vi "Day 2 Task 2.vi"() -> ()   [LabVIEW 2018]
panel:
  out "aim":i64
  out "Horizontal * vertical (multiplied)":i64
  out "vertical position":i64
  out "horizontal position":i64
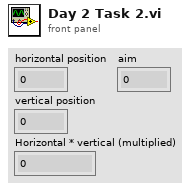
[diagram p1: front panel]
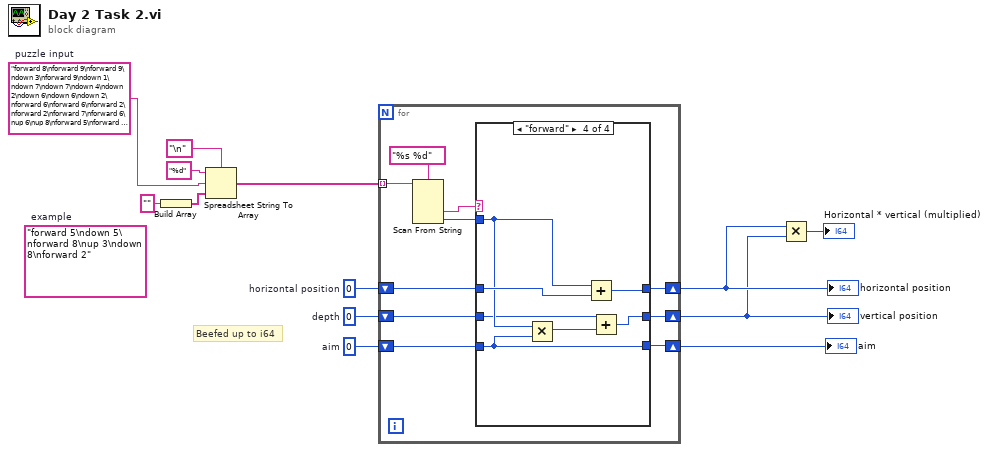
[diagram p0: block diagram]
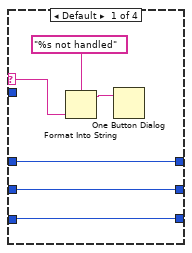
[diagram p2: hidden frame]
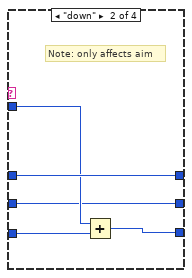
[diagram p3: hidden frame]
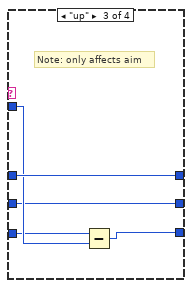
[diagram p4: hidden frame]
diagram:
  w3 = i64 0  # aim
  w1 = "forward 8\nforward 9\nforward 9\ndown 3\nforward 9\ndown 1\ndown 7\ndown 7\ndown 4\ndown 2\ndown 6\ndown 6\ndown 2\nforward 6\nforward 6\nforward 2\nforward 2\nforward 7\nforward 6\nup 6\nup 8\nforward 5\nforward 4\ndown 6\nforward 7\ndown 5\nforward 5\ndown 8\ndown 8\ndown 7\nforward 4\ndown 2\nforward 7\nup 8\nforward 3\ndown 2\nforward 1\nup 3\nforward 3\nup 1\ndown 3\nup 7\nup 2\ndown 4\ndown 2\nforward 9\nforward 3\ndown 8\nforward 5\nup 9\nup 4\nforward 9\ndown 1\nforward 6\ndown 3\nforward 8\nup 2\nforward 3\nup 7\ndown 4\nforward 2\nforward 7\nforward 3\ndown 1\ndown 3\nup 5\nforward 6\ndown 5\ndown 4\ndown 8\ndown 2\nup 5\nforward 7\nup 8\nforward 2\ndown 5\nforward 3\nup 1\nup 5\ndown 8\ndown 3\nforward 4\nforward 4\nforward 1\nup 8\ndown 9\nforward 7\nforward 9\ndown 5\nup 3\ndown 9\nup 6\nforward 1\nforward 3\nforward 5\ndown 5\nforward 6\ndown 3\ndown 8\nforward 3\nforward 5\nforward 7\nforward 6\ndown 9\ndown 5\ndown 6\ndown 5\ndown 1\ndown 8\nforward 3\ndown 9\ndown 5\ndown 5\nforward 9\nforward 2\ndown 7\nforward 9\nforward 9\nup 1\nforward 3\nup 9\nforward 5\nforward 7\ndown 7\nforward 2\nup 8\nup 6\ndown 7\ndown 3\ndown 5\ndown 2\nforward 6\nforward 6\nup 6\nup 2\nforward 4\nforward 7\nforward 1\ndown 4\nup 8\ndown 3\nup 1\ndown 2\nforward 4\nforward 7\nup 1\ndown 7\nforward 8\nup 2\ndown 8\nup 4\nup 4\nup 2\ndown 8\nup 4\ndown 6\nup 8\ndown 5\nup 5\ndown 8\nforward 9\ndown 1\ndown 5\nforward 3\nforward 3\nup 9\ndown 2\nforward 3\ndown 6\nforward 1\nforward 9\nforward 3\ndown 8\nup 4\ndown 1\ndown 8\nup 1\nforward 2\ndown 7\nup 3\nup 8\ndown 2\nup 6\nforward 6\ndown 9\nforward 4\nforward 7\nup 9\nforward 3\nforward 2\ndown 8\ndown 2\ndown 5\ndown 5\ndown 1\nup 7\ndown 4\nforward 5\ndown 9\ndown 5\ndown 1\ndown 6\nforward 9\ndown 6\nforward 3\ndown 3\nup 6\nforward 2\nforward 6\ndown 2\ndown 9\ndown 6\ndown 1\ndown 7\ndown 6\ndown 6\nup 1\nforward 8\ndown 9\ndown 6\ndown 8\ndown 8\ndown 6\ndown 3\nforward 9\nforward 6\ndown 9\nforward 5\ndown 6\ndown 6\ndown 9\ndown 7\ndown 3\nforward 1\nup 9\nforward 9\ndown 7\nforward 4\ndown 1\nforward 9\nup 9\ndown 7\nforward 5\ndown 3\nup 7\nforward 9\nforward 6\nforward 3\nforward 8\ndown 4\ndown 1\ndown 7\ndown 7\nup 4\ndown 9\nforward 6\nforward 7\ndown 8\nforward 2\nforward 2\nforward 9\nforward 6\nforward 9\nup 6\nup 8\nforward 2\nup 3\nforward 9\nforward 1\ndown 4\nforward 8\ndown 4\nforward 5\nforward 7\nup 2\nforward 5\ndown 4\nforward 3\ndown 5\nforward 9\nup 3\nforward 8\ndown 7\ndown 7\ndown 9\nforward 2\ndown 1\ndown 6\nup 8\ndown 2\ndown 1\nup 3\ndown 3\nforward 2\nforward 6\nup 6\ndown 3\nup 9\nup 3\ndown 8\nup 6\ndown 2\nforward 4\nup 1\ndown 5\ndown 4\nup 9\nup 7\nforward 7\ndown 9\nforward 9\nforward 5\nforward 3\ndown 4\nup 6\nup 7\ndown 7\ndown 6\nup 9\nup 4\ndown 7\nforward 7\nforward 8\ndown 9\nforward 5\nforward 4\ndown 5\nforward 8\nforward 5\nup 3\ndown 9\nforward 1\nforward 2\nup 3\ndown 2\ndown 1\nforward 5\nforward 5\nforward 6\nup 2\nforward 3\ndown 7\ndown 6\nup 3\ndown 4\ndown 4\nforward 5\ndown 3\nup 6\nforward 1\nup 8\nforward 7\nforward 1\nforward 9\ndown 2\nup 8\nup 1\nup 4\nforward 9\nforward 3\nforward 5\ndown 1\nup 9\ndown 1\nforward 3\ndown 6\ndown 8\nup 4\nforward 6\nup 7\ndown 8\nforward 9\nup 2\ndown 7\ndown 1\nforward 9\nup 7\nforward 3\nforward 9\nforward 1\nforward 1\ndown 9\nforward 1\nup 4\ndown 5\nforward 4\ndown 1\nforward 4\nforward 9\nup 4\ndown 3\ndown 6\nup 2\ndown 6\ndown 5\nforward 5\nup 1\nup 9\nforward 8\nup 3\ndown 1\nforward 3\nforward 7\nup 6\nup 3\ndown 6\nforward 7\nup 6\ndown 7\nforward 8\nup 4\ndown 8\nup 9\nup 3\ndown 3\nforward 8\ndown 4\ndown 9\nforward 2\ndown 7\nup 1\nforward 9\nforward 5\nup 8\nforward 9\nforward 4\nforward 9\nforward 7\ndown 4\nup 4\ndown 7\ndown 4\ndown 4\ndown 1\nforward 5\nforward 4\ndown 1\ndown 4\ndown 8\ndown 3\nforward 7\nforward 4\ndown 1\ndown 9\nup 3\nforward 2\ndown 8\ndown 9\ndown 2\ndown 5\nup 9\ndown 9\nup 9\nforward 5\nforward 8\nforward 9\ndown 5\nforward 6\ndown 8\ndown 9\nforward 8\nup 5\nup 9\nup 7\nup 8\nforward 9\nforward 1\nup 6\ndown 8\ndown 8\nforward 1\nup 1\nforward 8\nforward 6\ndown 4\nforward 1\ndown 7\nforward 8\nforward 3\nup 3\ndown 4\ndown 2\nforward 2\nforward 3\nup 4\ndown 3\nforward 2\ndown 8\nforward 7\nup 3\ndown 2\nforward 2\ndown 5\nup 6\nup 6\nforward 4\nup 4\ndown 8\nforward 8\ndown 9\ndown 9\ndown 6\ndown 2\nforward 2\nup 6\nup 5\nforward 3\nforward 3\nup 9\ndown 3\nforward 8\ndown 5\nforward 5\nforward 7\ndown 3\ndown 4\ndown 1\ndown 8\ndown 1\ndown 1\nforward 9\nforward 3\ndown 8\ndown 6\nup 9\nforward 1\nforward 5\nup 9\nup 8\nforward 2\nup 8\ndown 9\nup 2\nforward 5\nforward 1\nforward 8\ndown 3\nforward 4\ndown 5\nup 6\nforward 8\nforward 9\nforward 3\ndown 1\ndown 3\ndown 3\nup 4\nforward 9\ndown 3\ndown 6\nforward 3\nforward 2\ndown 6\ndown 8\nforward 6\nup 8\nup 3\nup 4\nforward 2\nforward 4\nforward 4\nforward 7\ndown 6\nup 8\ndown 3\nforward 8\nforward 4\ndown 7\ndown 5\nforward 6\nforward 4\nforward 6\ndown 3\nforward 3\ndown 1\ndown 7\nforward 3\nforward 2\nforward 7\ndown 5\nup 4\ndown 6\ndown 9\nforward 3\nforward 5\nforward 3\ndown 1\nforward 2\nup 5\nup 6\nforward 2\ndown 4\nforward 3\ndown 4\ndown 1\nforward 8\nup 2\ndown 3\ndown 6\nup 5\nforward 3\nforward 6\ndown 3\nforward 1\ndown 7\nforward 2\nforward 1\nforward 6\nforward 5\nforward 3\ndown 4\ndown 8\nforward 1\nup 2\nup 8\ndown 4\nforward 9\nup 6\nforward 5\nforward 7\ndown 5\nforward 5\ndown 1\nforward 4\nforward 5\nup 2\nforward 5\nup 8\nup 1\nforward 2\ndown 4\ndown 6\nforward 4\ndown 2\ndown 3\nforward 2\nup 3\nup 4\nforward 2\ndown 6\nforward 1\nforward 4\ndown 6\nforward 7\nup 2\nforward 7\nforward 6\nup 2\nforward 8\nforward 4\nforward 9\ndown 1\ndown 8\nforward 3\nforward 2\ndown 8\nup 1\nforward 4\ndown 8\nforward 2\nforward 8\nup 2\ndown 1\nforward 4\nforward 2\nup 4\nup 2\ndown 3\nup 8\nforward 3\nup 8\nforward 9\nup 1\nup 5\ndown 5\ndown 6\nforward 1\nup 5\nup 8\nforward 7\ndown 5\nup 4\nforward 2\nup 4\nup 4\ndown 2\nforward 6\nforward 2\ndown 7\ndown 5\nforward 1\ndown 2\ndown 5\ndown 7\nup 8\ndown 8\nup 5\ndown 1\nforward 5\ndown 2\nforward 5\ndown 1\nup 7\nup 2\nforward 2\nforward 3\nforward 6\nforward 3\ndown 8\nup 8\nforward 8\nforward 1\nforward 7\nup 2\nforward 9\ndown 1\nforward 5\nup 9\nforward 3\nforward 7\nforward 8\nup 1\ndown 3\nforward 5\ndown 2\nforward 6\nforward 3\ndown 9\nup 5\nforward 2\ndown 4\nup 1\nforward 4\nup 4\ndown 8\ndown 8\nforward 3\nforward 8\ndown 7\nup 3\nforward 1\nup 3\nforward 9\nforward 7\nforward 1\ndown 6\nforward 3\ndown 1\ndown 8\nforward 5\nforward 3\nup 6\nforward 5\nforward 4\nforward 3\nforward 9\nforward 8\ndown 6\ndown 2\nforward 7\nforward 6\nup 6\ndown 6\ndown 4\ndown 3\nforward 8\ndown 9\nup 5\nforward 3\nforward 2\ndown 5\nup 4\ndown 6\ndown 3\nforward 9\ndown 2\nforward 9\nforward 8\nup 1\ndown 2\nforward 7\nup 5\nup 6\ndown 8\nup 9\nup 8\nforward 1\nforward 5\ndown 9\nforward 8\ndown 8\nup 1\ndown 7\nforward 7\nup 3\ndown 3\ndown 1\nforward 2\ndown 3\nforward 9\nforward 2\ndown 8\ndown 2\nforward 5\ndown 9\ndown 1\ndown 5\ndown 6\nup 4\nup 3\ndown 1\nup 7\nforward 6\ndown 3\ndown 6\nup 5\nforward 8\nup 8\ndown 1\ndown 2\nup 8\ndown 7\nforward 7\nforward 4\ndown 8\ndown 3\nforward 3\ndown 4\nforward 3\ndown 6\nforward 4\nforward 7\nforward 9\nup 7\nforward 1\ndown 7\ndown 8\ndown 8\nup 6\ndown 3\nforward 5\nforward 5\nforward 9\nforward 4\ndown 4\ndown 8\ndown 7\ndown 1\nforward 2\nforward 4\ndown 3\ndown 6\ndown 7\nforward 5\ndown 8\ndown 1\nforward 4\nforward 3\nforward 1\ndown 6\ndown 7\ndown 1\nforward 6\ndown 4\nup 2\nforward 4\ndown 2\nup 5\ndown 2\ndown 6\nup 7\nforward 4\nforward 7\nforward 9\nup 5\ndown 9\nup 5\nforward 6\ndown 2\nup 8\nup 9\nup 9\nforward 5\ndown 2\nforward 2\ndown 7\nforward 5\nforward 9\nup 8\ndown 8\nforward 1\ndown 2\nup 3\nforward 3\ndown 5\nforward 4\ndown 3\nforward 4\nforward 9\nforward 3\ndown 5\nforward 4\ndown 2\nforward 5\nforward 8\nup 6\nup 2\ndown 3\nforward 6\ndown 5\ndown 4\ndown 4\ndown 4\nup 2\nup 2\nforward 6\nforward 2\nforward 9\ndown 2\ndown 9\ndown 8\nforward 2\ndown 3\nup 3\nforward 5\ndown 4\nup 3\nforward 3\ndown 1\nforward 7\nforward 5\nforward 6\ndown 8\ndown 5\ndown 5\ndown 9\nup 2\nforward 3\ndown 4\ndown 9\nforward 3\nforward 9\nforward 2\nforward 4\nup 6\ndown 6\nup 9\nforward 8\ndown 7\nforward 1\nforward 4\nup 1\nup 2\ndown 9\nforward 6\ndown 6\ndown 1\ndown 4\ndown 7\ndown 6\nforward 5\nup 1\nup 7\ndown 2\ndown 8\ndown 2\ndown 7\ndown 3\nup 9\ndown 7\ndown 5\ndown 6\nforward 9\nup 3\nforward 2\ndown 8\nforward 4\ndown 6\nforward 3\nup 3\ndown 5\nup 4\nforward 6\nforward 7\nforward 9\ndown 3\nforward 7\nforward 3\ndown 4\nup 4\ndown 8\nforward 6\nforward 7\nforward 9\nforward 4\ndown 3\nup 5\ndown 7\ndown 7\nforward 9"  # puzzle input
  w7 = i64 0  # depth
  w8 = i64 0  # horizontal position
  (unwired) "forward 5\ndown 5\nforward 8\nup 3\ndown 8\nforward 2"  # example
  # "Beefed up to i64"
  n1 = Build Array("") -> (w11:string[])
  n2 = Spreadsheet String To Array(delimiter (Tab)="\n", format string="%d", spreadsheet string=w1, array type (2D Dbl)=w11) -> (array=w9:string[])
  n3 = for {
    tunnel: w9 -> [w21] mode=indexing
    shift-right: [w20] -> w6
    shift-left: w8 -> [w19]
    shift-right: [w17] -> w5
    shift-left: w7 -> [w18]
    shift-right: [w14] -> w2
    shift-left: w3 -> [w15]
    n4 = Scan From String(format string="%s %d", input string=w21) -> (output 1=w22:string, output 2=w16:i32)  [unwired: 4 in, 3 out]
    n5 = case shown="\"forward\"" w22 {
      selector: w22 -> [w27 _ _ _]
      tunnel: [w29 w34 w39 w45] -> w20
      tunnel: w19 -> [w29 w34 w39 w46]
      tunnel: w18 -> [w28 w30 w35 w41]
      tunnel: [w28 w30 w35 w40] -> w17
      tunnel: w16 -> [_ w33 w38 w43]
      tunnel: w15 -> [w24 w32 w37 w44]
      tunnel: [w24 w31 w36 w44] -> w14
      frame Default {
        n6 = Format Into String(format string="%s not handled", w27) -> (resulting string=w26:string)  [unwired: 2 in, 1 out]
        n7 = One Button Dialog(message=w26) -> ()  [unwired: 1 in, 1 out]
      }
      frame "down" {
        # "Note: only affects aim"
        n8 = Add(x=w33, y=w32) -> (x+y=w31:i64)
      }
      frame "up" {
        # "Note: only affects aim"
        n9 = Subtract(x=w37, y=w38) -> (x-y=w36:i64)
      }
      frame "forward" {
        n10 = Multiply(x=w43, y=w44) -> (x*y=w42:i64)
        n11 = Add(x=w43, y=w46) -> (x+y=w45:i64)
        n12 = Add(x=w41, y=w42) -> (x+y=w40:i64)
      }
    }
  }
  "horizontal position" <- w6
  "vertical position" <- w5
  "aim" <- w2
  n13 = Multiply(x=w6, y=w5) -> (x*y=→"Horizontal * vertical (multiplied)":i64)
